vi "PolarizePodStateData.vi"(11 "Pod State Data":T1) -> (3 "Normalized, polarized state data":T1)   [LabVIEW 2014]
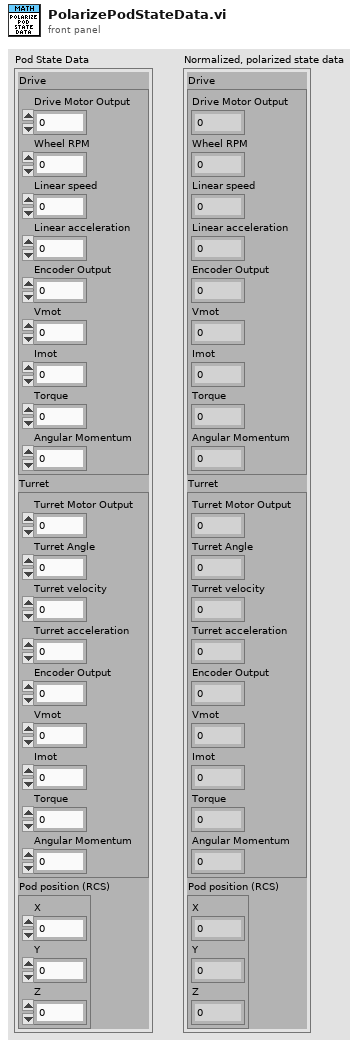
[diagram p1: front panel]
types:
  T1 = cluster{"Drive":cluster{"Drive Motor Output":dbl, "Wheel RPM":dbl, "Linear speed":dbl, "Linear acceleration":dbl, "Encoder Output":dbl, "Vmot":dbl, "Imot":dbl, "Torque":dbl, "Angular Momentum":dbl}, "Turret":cluster{"Turret Motor Output":dbl, "Turret Angle":dbl, "Turret velocity":dbl, "Turret acceleration":dbl, "Encoder Output":dbl, "Vmot":dbl, "Imot":dbl, "Torque":dbl, "Angular Momentum":dbl}, "Pod position (RCS)":cluster{"X":dbl, "Y":dbl, "Z":dbl}}
  T2 = cluster{"Drive Motor Output":dbl, "Wheel RPM":dbl, "Linear speed":dbl, "Linear acceleration":dbl, "Encoder Output":dbl, "Vmot":dbl, "Imot":dbl, "Torque":dbl, "Angular Momentum":dbl}
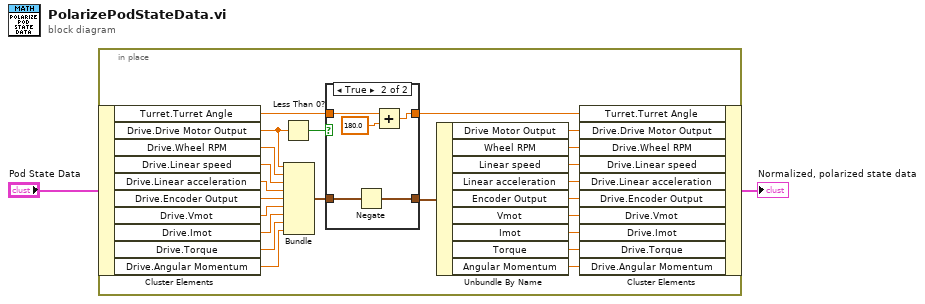
[diagram p0: block diagram]
diagram:
  n1 = in-place {
    n2 = in-place-cluster #1("Pod State Data") -> ("Turret.Turret Angle"=w24:dbl, "Drive.Drive Motor Output"=w22:dbl, "Drive.Wheel RPM"=w21:dbl, "Drive.Linear speed"=w20:dbl, "Drive.Linear acceleration"=w19:dbl, "Drive.Encoder Output"=w18:dbl, "Drive.Vmot"=w17:dbl, "Drive.Imot"=w14:dbl, "Drive.Torque"=w15:dbl, "Drive.Angular Momentum"=w16:dbl)
    n3 = Less Than 0?(x=w22) -> (x < 0?=w25:bool)
    n4 = Bundle("Drive Motor Output"=w22, "Wheel RPM"=w21, "Linear speed"=w20, "Linear acceleration"=w19, "Encoder Output"=w18, "Vmot"=w17, "Imot"=w14, "Torque"=w15, "Angular Momentum"=w16) -> (w13:T2)  [unwired: 1 in]
    n5 = case shown="True" w25 {
      tunnel: [w27 w32] -> w23
      tunnel: w24 -> [w27 w31]
      tunnel: w13 -> [w26 w30]
      tunnel: [w26 w29] -> w12
      frame False {
      }
      frame True {
        n6 = Negate(x=w30) -> (-x=w29:T2)
        n7 = Add(x=w31, y=180.0) -> (x+y=w32:dbl)
      }
    }
    n8 = Unbundle By Name(w12) -> ("Drive Motor Output"=w11:dbl, "Wheel RPM"=w10:dbl, "Linear speed"=w9:dbl, "Linear acceleration"=w8:dbl, "Encoder Output"=w7:dbl, "Vmot"=w6:dbl, "Imot"=w5:dbl, "Torque"=w4:dbl, "Angular Momentum"=w3:dbl)
    n9 = in-place-cluster #1("Turret.Turret Angle"=w23, "Drive.Drive Motor Output"=w11, "Drive.Wheel RPM"=w10, "Drive.Linear speed"=w9, "Drive.Linear acceleration"=w8, "Drive.Encoder Output"=w7, "Drive.Vmot"=w6, "Drive.Imot"=w5, "Drive.Torque"=w4, "Drive.Angular Momentum"=w3) -> (→"Normalized, polarized state data":T1)
  }
